vi "FGV_GraphData.vi"(7 "Mode":enum16{"Reset", "Add", "Get"}(ring), 8 "error in (no error)":errorcluster, 11 "Data":T1[](array[typedef])) -> (0 "error out":errorcluster, 3 "Data out":T1[](array[typedef]))   [LabVIEW 2020]
uses:
  <vilib>/Stadlmann TEC/OXYGEN Datastream/VIs/Data Aquasation/TypeDefs/DataPoint_Double.ctl
  <vilib>/Stadlmann TEC/OXYGEN Datastream/OXYGEN_Datastream.lvlib
  VIs/editGraphData.vi
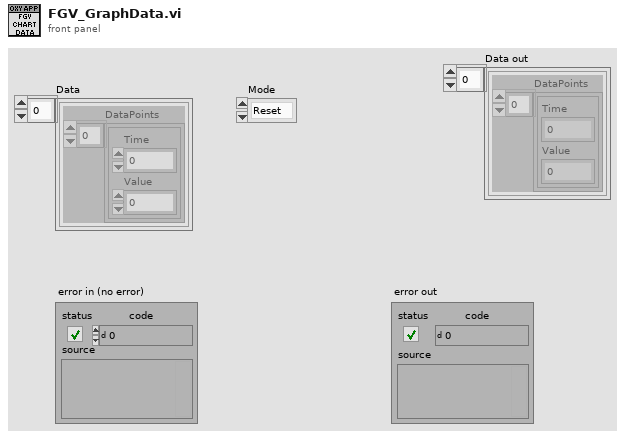
[diagram p1: front panel]
types:
  T1 = typedef "OXYGEN_Datastream.lvlib/DataPoint_Double.ctl" = cluster{"DataPoints":cluster{"Time":dbl, "Value":dbl}[]}
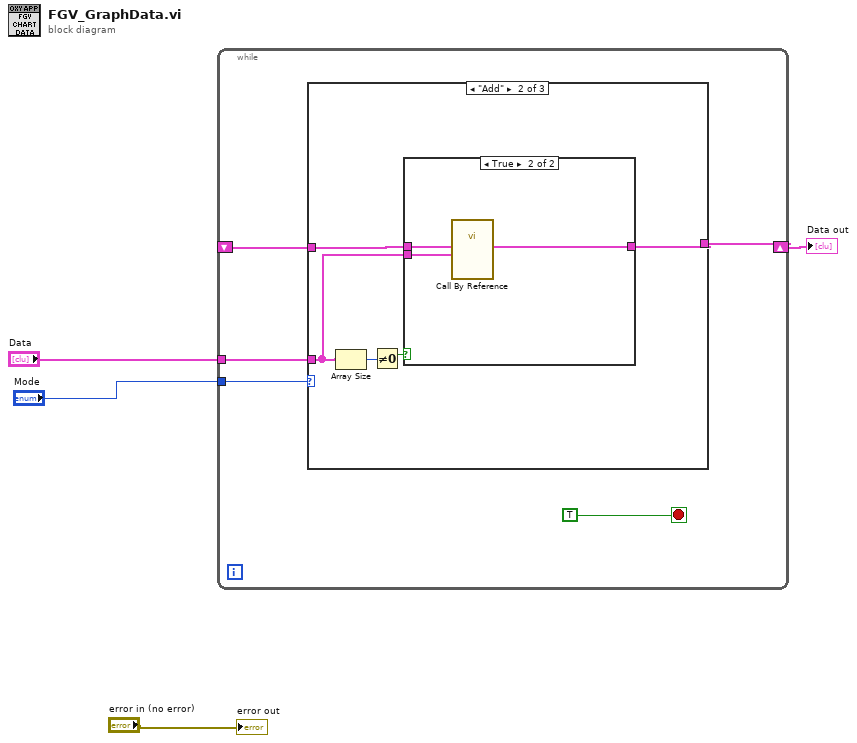
[diagram p0: block diagram]
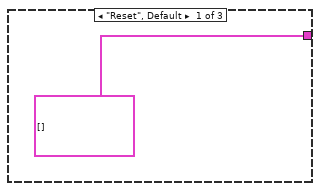
[diagram p2: hidden frame]
diagram:
  n1 = while {
    tunnel: "Mode" -> [w8]
    tunnel: "Data" -> [w7]
    shift-right: [w5] -> w1
    shift-left: _ -> [w6]
    stop <- TRUE stop-if-true
    n2 = case shown="\"Add\"" w8 {
      tunnel: w7 -> [_ w13 _]
      tunnel: [T1[] [] ("Data") w15 w20] -> w5
      tunnel: w6 -> [_ w14 w20]
      frame "Reset", Default {
      }
      frame "Add" {
        n3 = Array Size(array=w13) -> (size(s)=w12:i32)
        n4 = Not Equal To 0?(x=w12) -> (x != 0?=w11:bool)
        n5 = case shown="True" w11 {
          tunnel: [w16 w19] -> w15
          tunnel: w13 -> [_ w18]
          tunnel: w14 -> [w16 w17]
          frame False {
          }
          frame True {
            n6 = call-by-ref "?"("Data 2"=w18, "Data"=w17) -> ("Data 3"=w19:T1[])  [unwired: 10 in, 3 out]
          }
        }
      }
      frame "Get" {
      }
    }
  }
  "Data out" <- w1
  "error out" <- "error in (no error)"
